vi "testSendTelMultiple.vi"(8 "error in (no error)":errorcluster) -> (0 "error out":errorcluster)   [LabVIEW 2018]
uses:
  src/TcpServer/TcpServer.lvclass
  src/TcpServerTel/typedef/telTypeDef.ctl
  <vilib>/addons/_JKI Toolkits/Caraya/classes/Assert/Assert Equal Value_Variant.vi
  <vilib>/addons/_JKI Toolkits/Caraya/classes/Test/Test.lvclass
  <vilib>/addons/_JKI Toolkits/Caraya/classes/Assert/Assert.lvclass
  src/TcpServerTel/TcpServerTel.lvclass
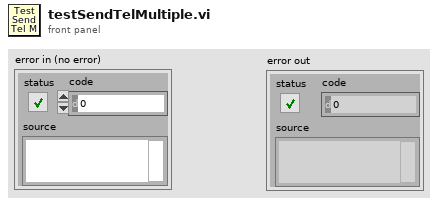
[diagram p1: front panel]
types:
  T1 = typedef "TcpServerTel.lvclass/telTypeDef.ctl" = cluster{"name":string, "telDetails":string}
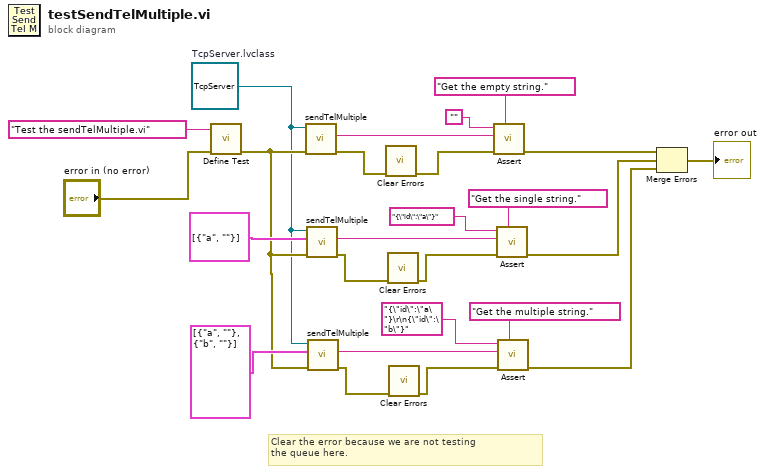
[diagram p0: block diagram]
diagram:
  w2 = refnum<class "TcpServer.lvclass"> refnum  # TcpServer.lvclass
  # "Clear the error because we are not testing\nthe queue here."
  n1 = call <vilib>:"Define Test.vi"("error in (no error)"="error in (no error)", "Label (VI Title)"="Test the sendTelMultiple.vi") -> ("error out"=w7:errorcluster)  [unwired: 8 in, 1 out]
  n2 = call "sendTelMultiple.vi"("error in (no error)"=w7, "TcpServer in"=w2) -> ("error out"=w23:errorcluster, "string"=w21:string)  [unwired: 7 in, 1 out]
  n3 = call "sendTelMultiple.vi"("error in (no error)"=w7, "telemetry"=T1[] [{"name"="a", "telDetails"=""}], "TcpServer in"=w2) -> ("error out"=w16:errorcluster, "string"=w17:string)  [unwired: 6 in, 1 out]
  n4 = call "sendTelMultiple.vi"("error in (no error)"=w7, "telemetry"=T1[] [{"name"="a", "telDetails"=""}, {"name"="b", "telDetails"=""}], "TcpServer in"=w2) -> ("error out"=w10:errorcluster, "string"=w11:string)  [unwired: 6 in, 1 out]
  n5 = call <vilib>:"Clear Errors.vi"("error in (no error)"=w23) -> ("error out"=w22:errorcluster)  [unwired: 5 in, 1 out]
  n6 = call <vilib>:"Clear Errors.vi"("error in (no error)"=w16) -> ("error out"=w15:errorcluster)  [unwired: 5 in, 1 out]
  n7 = call <vilib>:"Clear Errors.vi"("error in (no error)"=w10) -> ("error out"=w9:errorcluster)  [unwired: 5 in, 1 out]
  n8 = call-poly <vilib>:"Assert.vi"("Label"="Get the empty string.", "error in (no error)"=w22, "Y"=w21, "X"="") -> ("error out"=w6:errorcluster)  [unwired: 6 in, 1 out]
  n9 = call-poly <vilib>:"Assert.vi"("Label"="Get the single string.", "error in (no error)"=w15, "Y"=w17, "X"="{\"id\":\"a\"}") -> ("error out"=w5:errorcluster)  [unwired: 6 in, 1 out]
  n10 = call-poly <vilib>:"Assert.vi"("Label"="Get the multiple string.", "error in (no error)"=w9, "Y"=w11, "X"="{\"id\":\"a\"}\r\n{\"id\":\"b\"}") -> ("error out"=w4:errorcluster)  [unwired: 6 in, 1 out]
  n11 = Merge Errors(w6, w5, w4) -> (→"error out":errorcluster)
